vi "Mono SubVI Test Structure.vi"() -> ()   [LabVIEW 2017]
uses:
  C:/Users/Admin/Desktop/connection test/Cornerstone.dll
  Cornerstone.dll
panel:
  out "getWavelength":dbl
  out "Wavelength Set?":bool=TRUE
  in  "Wavelength":dbl format="%#_13g"
  out ".NET Refnum":refnum<k24>
  out "error out":errorcluster
  in  "error in (no error)":errorcluster
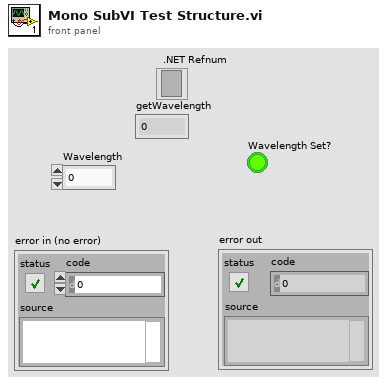
[diagram p1: front panel]
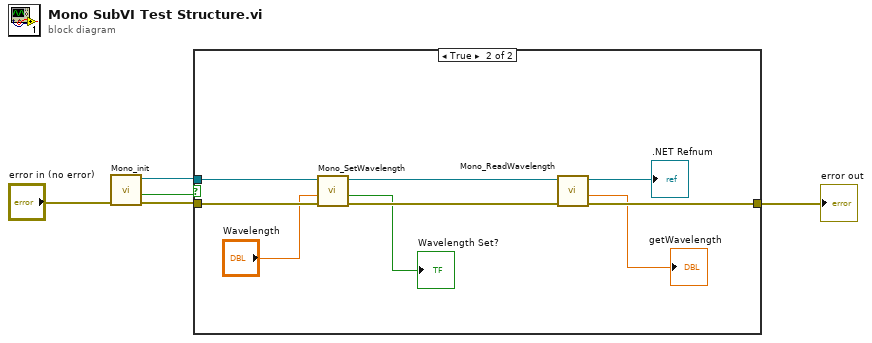
[diagram p0: block diagram]
diagram:
  n1 = call "Mono_init.vi"("error in (no error)"="error in (no error)") -> ("error out"=w5:errorcluster, "Mono Connected?"=w4:bool, "CmdLib"=w1:refnum<k24>)  [unwired: 8 in]
  n2 = case shown="True" w4 {
    tunnel: w5 -> [w6 w14]
    tunnel: [w6 w10] -> w2
    tunnel: w1 -> [_ w15]
    frame False {
    }
    frame True {
      n3 = call "Mono_SetWavelength.vi"("error in (no error) 2"=w14, "Wavelength"="Wavelength", "CmdLib In"=w15) -> ("error out 2"=w11:errorcluster, "Wavelength Set"=→"Wavelength Set?":bool, "CmdLib Out"=w12:refnum<k24>)  [unwired: 6 in]
      n4 = call "Mono_ReadWavelength.vi"("error in (no error) 2"=w11, "CmdLib In"=w12) -> ("error out 2"=w10:errorcluster, "getWavelength"=→"getWavelength":dbl, "CmdLib Out"=→".NET Refnum":refnum<k24>)  [unwired: 7 in]
    }
  }
  "error out" <- w2
